vi "Main.vi"() -> ()   [LabVIEW 2020]
doc: "This template is for the Queued Message Handler design pattern.\n\nThe Event Handling Loop generates messages based on user interface actions.\n\nThe Message Handling Loop processes messages generated by the Event Handling Loop, or by other messages. The messages are string values, so new messages can be added easily to the Message Cases case structure in the Message Handling Loop. Each message cluster can also provide an optional value for Message Data, which is a variant that can be converted to whatever message-specific data is required."
uses:
  controls/WashIndicators.ctl
  controls/WashOptions.ctl
  controls/UI Data.ctl
  support/Message Queue/Message Queue.lvlib
  support/User Event - Stop/User Event - Stop.lvlib
panel:
  out "Wash Entry 2":bool
  in  "Wash Options":T1
  out "Car Wash Indicators 2":T2
  in  "Car Position Slider":u16(slide) scale=0.0..4.0
  out "Elapsed Time":dbl format="%<%H:%M:%S>t"
  in  "Start":bool
  in  "Stop":bool
  # "Pre-Soak\nH-P Wash\nL-P Wax\nSpot Free Rinse"
  # "Underbody Wash\nBug Remover"
  # "Tire Shine\nAir Dry"
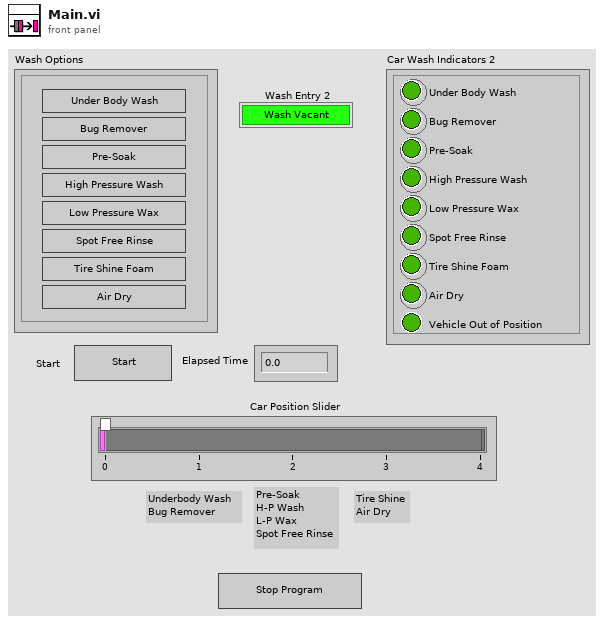
[diagram p1: front panel]
types:
  T1 = typedef "WashOptions.ctl" = cluster{"Bug Remover":bool, "Low Pressure Wax":bool, "High Pressure Wash":bool, "Pre-Soak":bool, "Spot Free Rinse":bool, "Air Dry":bool, "Under Body Wash":bool, "Tire Shine Foam":bool}
  T2 = typedef "WashIndicators.ctl" = cluster{"Bug Remover":bool, "Pre-Soak":bool, "High Pressure Wash":bool, "Spot Free Rinse":bool, "Tire Shine Foam":bool, "Low Pressure Wax":bool, "Vehicle Out of Position":bool, "Air Dry":bool, "Under Body Wash":bool}
  T3 = typedef "UI Data.ctl" = cluster{"Elapsed Time":refnum<vi>, "Car Position Slider":refnum<vi>, "Wash Options":refnum<vi>, "Car Wash Indicators 2":T2, "Wash Entry 2":bool}
  T4 = typedef "Message Queue.lvlib/All Message Queues.ctl" = cluster{"UI":refnum<queue>, "Status Loop":refnum<queue>}
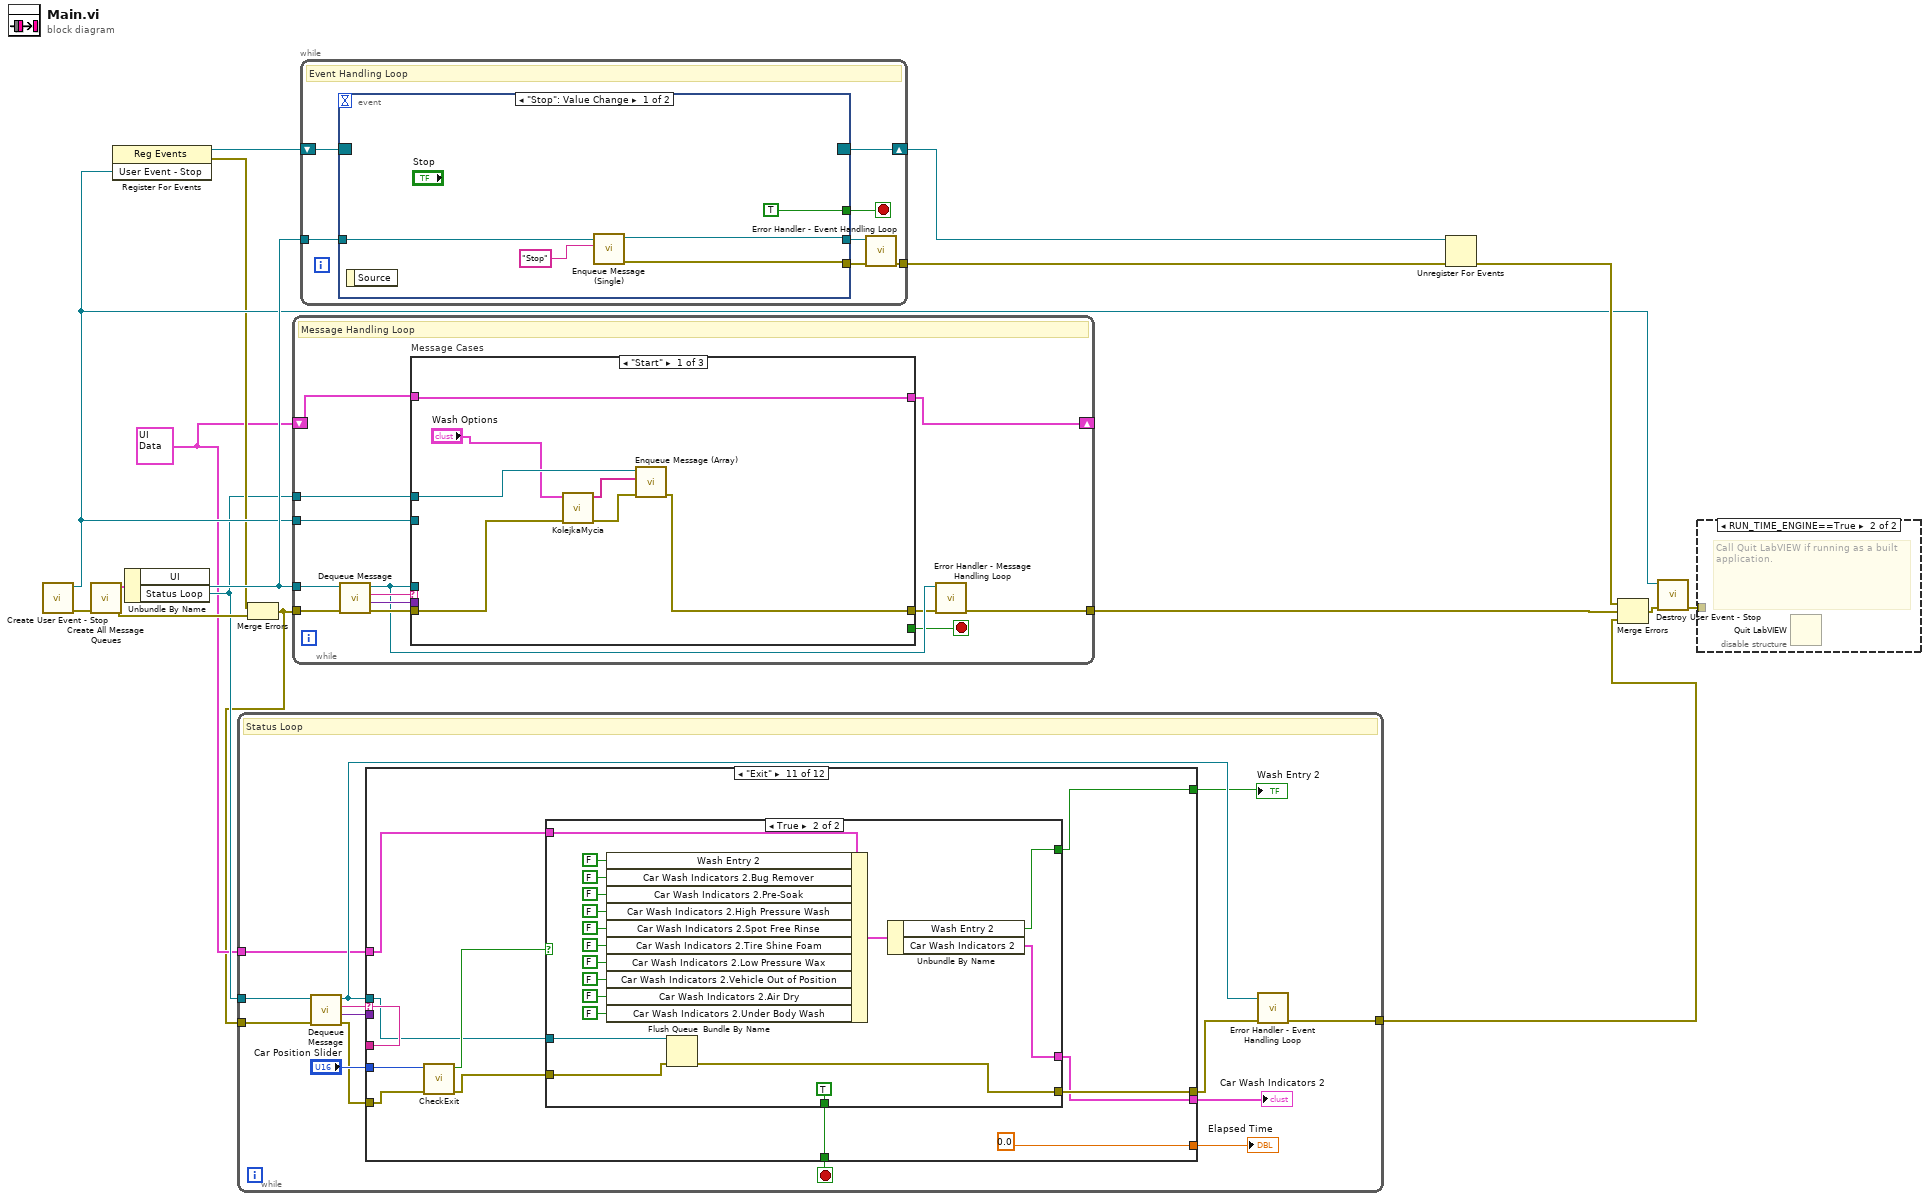
[diagram p0: block diagram]
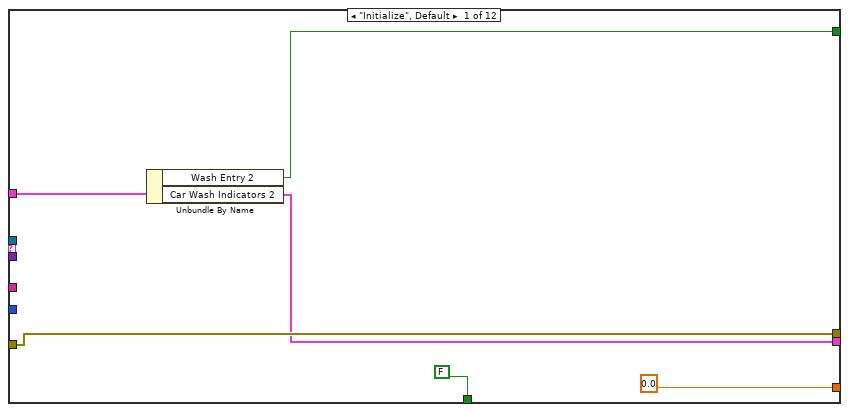
[diagram p2: hidden frame]
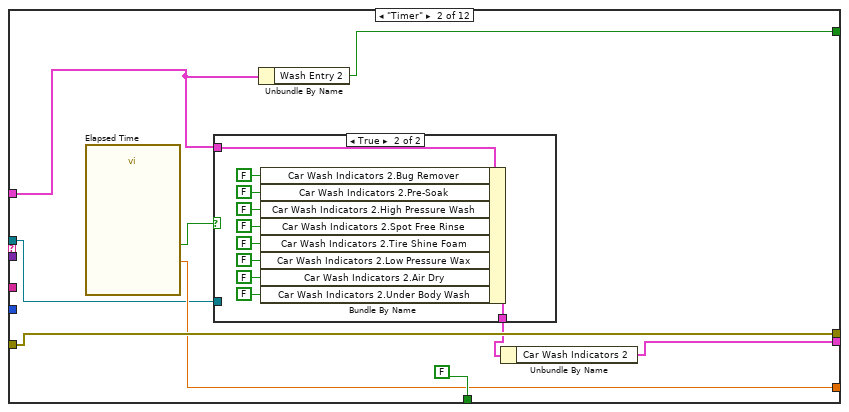
[diagram p3: hidden frame]
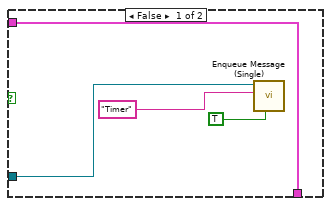
[diagram p4: hidden frame]
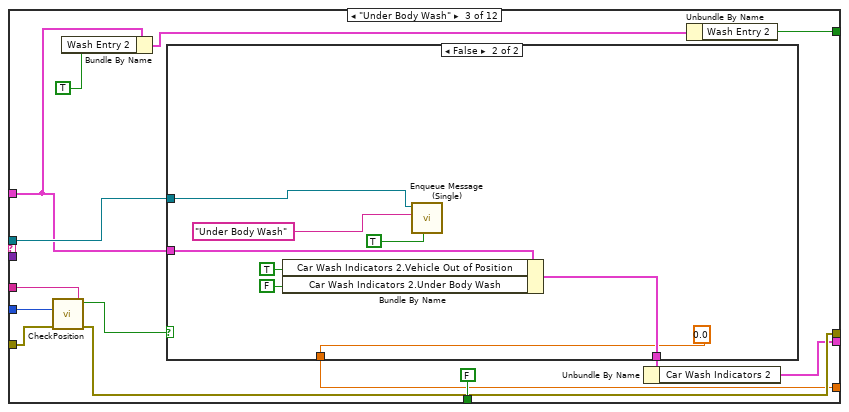
[diagram p5: hidden frame]
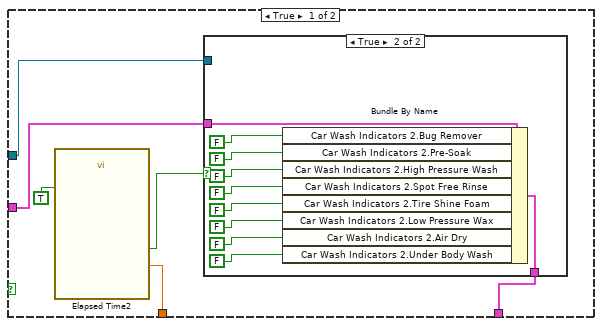
[diagram p6: hidden frame]
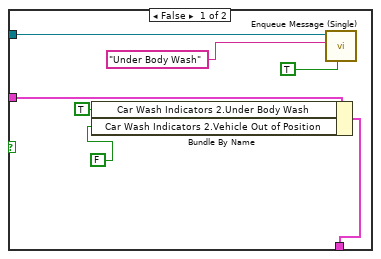
[diagram p7: hidden frame]
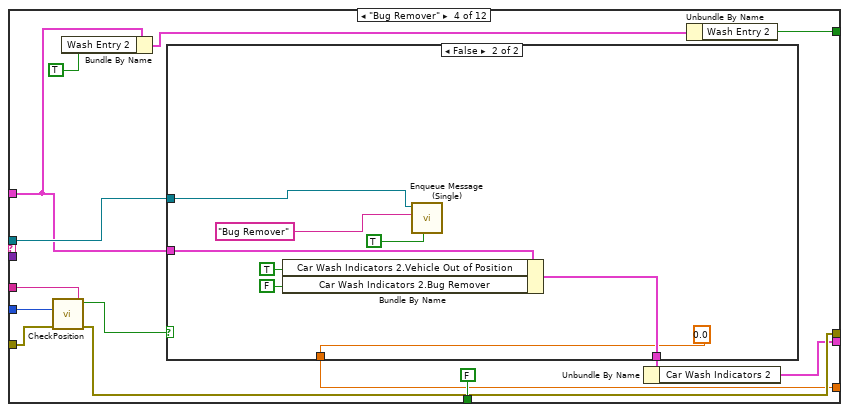
[diagram p8: hidden frame]
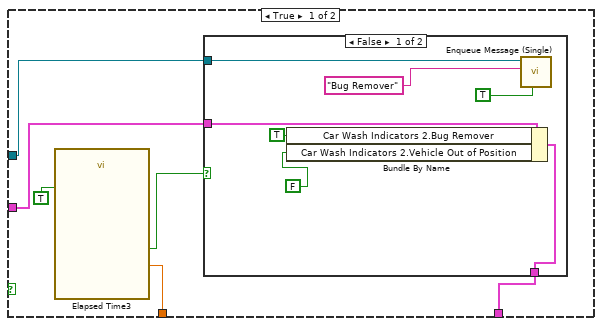
[diagram p9: hidden frame]
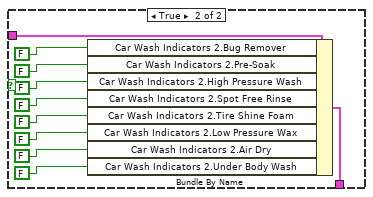
[diagram p10: hidden frame]
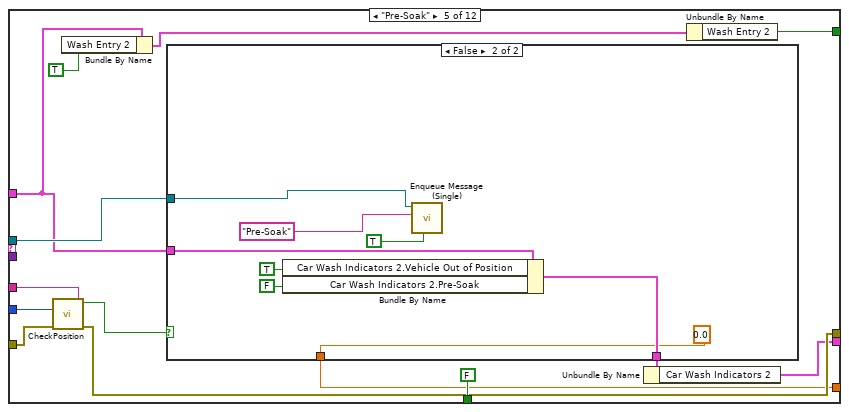
[diagram p11: hidden frame]
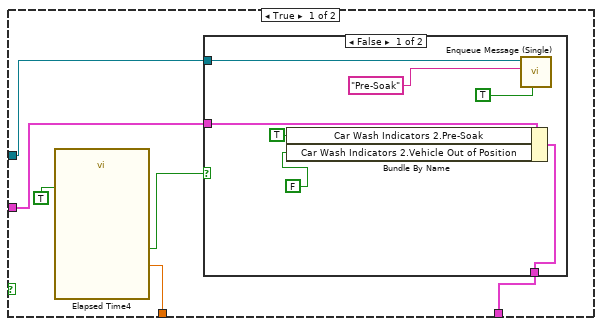
[diagram p12: hidden frame]
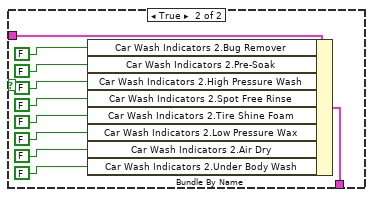
[diagram p13: hidden frame]
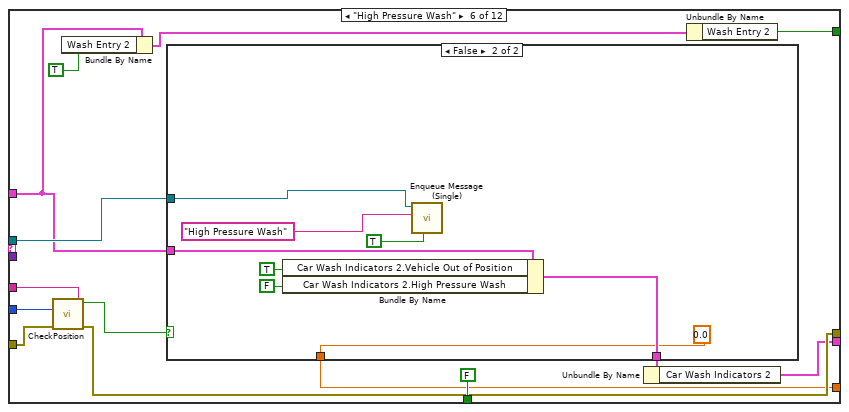
[diagram p14: hidden frame]
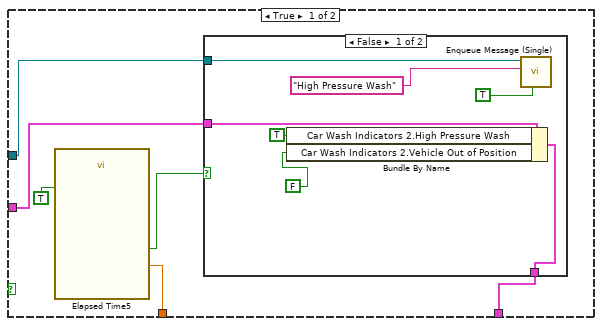
[diagram p15: hidden frame]
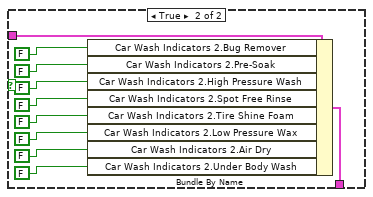
[diagram p16: hidden frame]
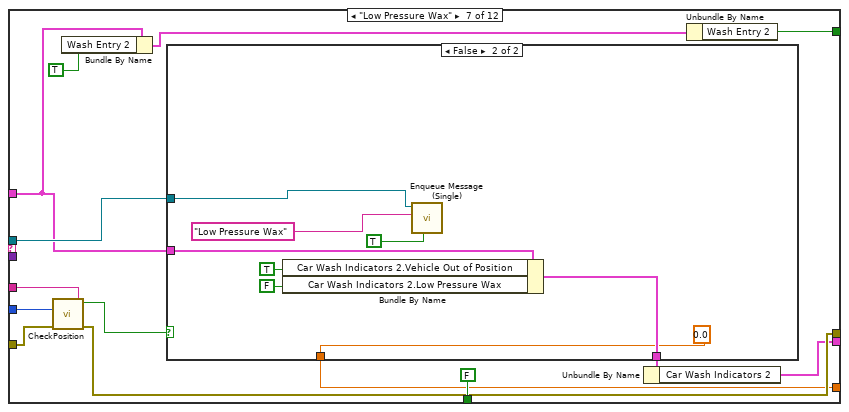
[diagram p17: hidden frame]
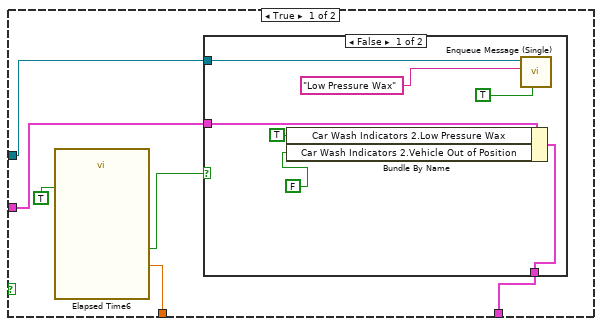
[diagram p18: hidden frame]
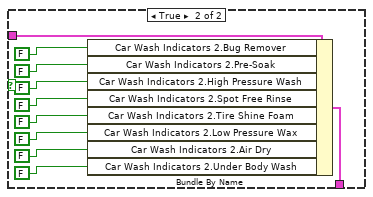
[diagram p19: hidden frame]
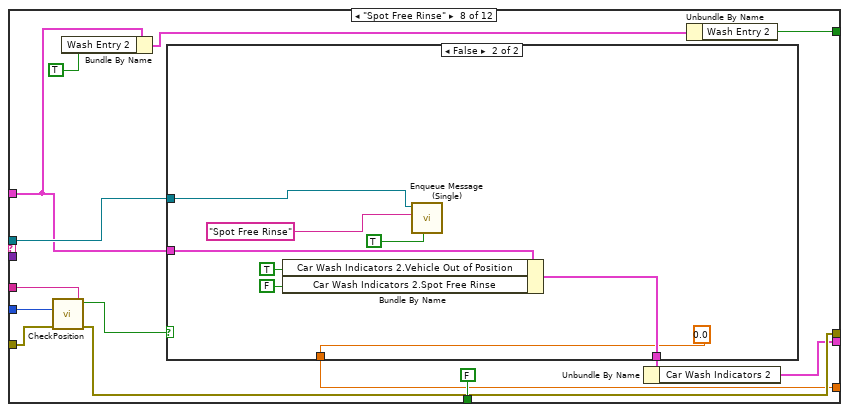
[diagram p20: hidden frame]
diagram:
  w2 = T3 {"Elapsed Time"=refnum, "Car Position Slider"=refnum, "Wash Options"=refnum, "Car Wash Indicators 2"={"Bug Remover"=FALSE, "Pre-Soak"=FALSE, "High Pressure Wash"=FALSE, "Spot Free Rinse"=FALSE, "Tire Shine Foam"=FALSE, "Low Pressure Wax"=FALSE, "Vehicle Out of Position"=FALSE, "Air Dry"=FALSE, "Under Body Wash"=FALSE}, "Wash Entry 2"=FALSE} ("Data Cluster")
  n1 = call "Create User Event - Stop.vi"() -> ("error out"=w13:errorcluster, "User Event - Stop"=w6:refnum<user-event>)  [unwired: 10 in]
  n2 = call "Create All Message Queues.vi"("error in (no error)"=w13) -> ("error out"=w17:errorcluster, "Message Queues out"=w16:T4)  [unwired: 9 in]
  n3 = register-events(w6) -> (reference out=w7:refnum<event-registration>, error out=w5:errorcluster)  [unwired: 2 in]
  n4 = Unbundle By Name(w16) -> ("UI"=w14:refnum<queue>, "Status Loop"=w3:refnum<queue>)
  n5 = Merge Errors(w5, w17) -> (w1:errorcluster)
  n6 = while {
    tunnel: w3 -> [w31]
    tunnel: w1 -> [w30]
    tunnel: [w27] -> w4
    tunnel: w2 -> [w25]
    stop <- w24 stop-if-true
    # "Status Loop"
    n7 = call "Dequeue Message.vi"("error in (no error)"=w30, "Message Queue"=w31) -> ("error out"=w21:errorcluster, "Message Data"=w29:variant, "Message"=w22:string, "dup Message Queue"=w26:refnum<queue>)  [unwired: 6 in]
    n8 = case shown="\"Exit\"" w22 {
      tunnel: w26 -> [_ w40 w69 w113 w158 w203 w248 w293 w338 w383 w425 w479]
      tunnel: w29 -> [_ _ _ _ _ _ _ _ _ _ _ _]
      tunnel: [w36 w45 w71 w115 w160 w205 w250 w295 w340 w385 w424 w482] -> w28
      tunnel: w25 -> [w35 w39 w65 w109 w154 w199 w244 w289 w334 w379 w423 w475]
      tunnel: [FALSE FALSE FALSE FALSE FALSE FALSE FALSE FALSE FALSE FALSE w426 TRUE] -> w24
      tunnel: "Car Position Slider" -> [_ _ w62 w117 w162 w207 w252 w297 w342 w387 w430 _]
      tunnel: w22 -> [_ _ w73 w118 w163 w208 w253 w298 w343 w388 _ _]
      tunnel: w21 -> [w36 w45 w72 w116 w161 w206 w251 w296 w341 w386 w429 w478]
      tunnel: [w34 w42 w67 w111 w156 w201 w246 w291 w336 w381 w421 w462] -> w20
      tunnel: [0.0 ("Elapsed Time (s)") w41 w66 w110 w155 w200 w245 w290 w335 w380 0.0 ("Elapsed Time (s)") 0.0 ("Elapsed Time (s)")] -> w19
      tunnel: [w32 w38 w63 w106 w151 w196 w241 w286 w331 w376 w422 w463] -> w18
      frame "Initialize", Default {
        n9 = Unbundle By Name(w35) -> ("Wash Entry 2"=w32:bool, "Car Wash Indicators 2"=w34:T2)
      }
      frame "Timer" {
        n10 = call "Elapsed Time"() -> ("Elapsed Time (s)"=w41:dbl, "Time has Elapsed"=w44:bool)  [unwired: 12 in, 6 out]
        n11 = case shown="True" w44 {
          tunnel: [w50 w52] -> w43
          tunnel: w39 -> [w50 w51]
          tunnel: w40 -> [w47 _]
          frame False {
            n12 = call "Enqueue Message (Single).vi"("Priority Message? (F)"=TRUE, "Message"="Timer", "Message Queue"=w47) -> ()  [unwired: 7 in, 2 out]
          }
          frame True {
            n13 = Bundle By Name(cluster=w51, "Car Wash Indicators 2.Bug Remover"=FALSE ("Bug Remover"), "Car Wash Indicators 2.Pre-Soak"=FALSE ("Pre-Soak"), "Car Wash Indicators 2.High Pressure Wash"=FALSE ("High Pressure Wash"), "Car Wash Indicators 2.Spot Free Rinse"=FALSE ("Spot Free Rinse"), "Car Wash Indicators 2.Tire Shine Foam"=FALSE ("Tire Shine Foam"), "Car Wash Indicators 2.Low Pressure Wax"=FALSE ("Low Pressure Wax"), "Car Wash Indicators 2.Air Dry"=FALSE ("Air Dry"), "Car Wash Indicators 2.Under Body Wash"=FALSE ("Under Body Wash")) -> (w52:T3)
          }
        }
        n14 = Unbundle By Name(w39) -> ("Wash Entry 2"=w38:bool)
        n15 = Unbundle By Name(w43) -> ("Car Wash Indicators 2"=w42:T2)
      }
      frame "Under Body Wash" {
        n16 = call "CheckPosition.vi"("error in"=w72, "Car Position"=w62, "State"=w73) -> ("error out"=w71:errorcluster, "Pozycja"=w70:bool)  [unwired: 7 in]
        n17 = Bundle By Name(cluster=w65, "Wash Entry 2"=TRUE) -> (w64:T3)
        n18 = case shown="False" w70 {
          tunnel: w65 -> [w76 w105]
          tunnel: w69 -> [w77 w102]
          tunnel: [w79 w99] -> w68
          tunnel: [w78 0.0 ("Elapsed Time (s)")] -> w66
          frame True {
            n19 = call "Elapsed Time2"("Auto Reset"=TRUE) -> ("Elapsed Time (s)"=w78:dbl, "Time has Elapsed"=w80:bool)  [unwired: 11 in, 6 out]
            n20 = case shown="True" w80 {
              tunnel: [w81 w89] -> w79
              tunnel: w77 -> [w85 _]
              tunnel: w76 -> [w84 w88]
              frame False {
                n21 = Bundle By Name(cluster=w84, "Car Wash Indicators 2.Under Body Wash"=TRUE, "Car Wash Indicators 2.Vehicle Out of Position"=FALSE) -> (w81:T3)
                n22 = call "Enqueue Message (Single).vi"("Priority Message? (F)"=TRUE, "Message"="Under Body Wash", "Message Queue"=w85) -> ()  [unwired: 7 in, 2 out]
              }
              frame True {
                n23 = Bundle By Name(cluster=w88, "Car Wash Indicators 2.Bug Remover"=FALSE ("Bug Remover"), "Car Wash Indicators 2.Pre-Soak"=FALSE ("Pre-Soak"), "Car Wash Indicators 2.High Pressure Wash"=FALSE ("High Pressure Wash"), "Car Wash Indicators 2.Spot Free Rinse"=FALSE ("Spot Free Rinse"), "Car Wash Indicators 2.Tire Shine Foam"=FALSE ("Tire Shine Foam"), "Car Wash Indicators 2.Low Pressure Wax"=FALSE ("Low Pressure Wax"), "Car Wash Indicators 2.Air Dry"=FALSE ("Air Dry"), "Car Wash Indicators 2.Under Body Wash"=FALSE ("Under Body Wash")) -> (w89:T3)
              }
            }
          }
          frame False {
            n24 = Bundle By Name(cluster=w105, "Car Wash Indicators 2.Vehicle Out of Position"=TRUE, "Car Wash Indicators 2.Under Body Wash"=FALSE) -> (w99:T3)
            n25 = call "Enqueue Message (Single).vi"("Priority Message? (F)"=TRUE, "Message"="Under Body Wash", "Message Queue"=w102) -> ()  [unwired: 7 in, 2 out]
          }
        }
        n26 = Unbundle By Name(w68) -> ("Car Wash Indicators 2"=w67:T2)
        n27 = Unbundle By Name(w64) -> ("Wash Entry 2"=w63:bool)
      }
      frame "Bug Remover" {
        n28 = call "CheckPosition.vi"("error in"=w116, "Car Position"=w117, "State"=w118) -> ("error out"=w115:errorcluster, "Pozycja"=w114:bool)  [unwired: 7 in]
        n29 = Bundle By Name(cluster=w109, "Wash Entry 2"=TRUE) -> (w107:T3)
        n30 = case shown="False" w114 {
          tunnel: w109 -> [w121 w150]
          tunnel: w113 -> [w122 w147]
          tunnel: [w124 w144] -> w112
          tunnel: [w123 0.0 ("Elapsed Time (s)")] -> w110
          frame True {
            n31 = call "Elapsed Time3"("Auto Reset"=TRUE) -> ("Elapsed Time (s)"=w123:dbl, "Time has Elapsed"=w125:bool)  [unwired: 11 in, 6 out]
            n32 = case shown="False" w125 {
              tunnel: [w126 w134] -> w124
              tunnel: w122 -> [w130 _]
              tunnel: w121 -> [w129 w133]
              frame False {
                n33 = Bundle By Name(cluster=w129, "Car Wash Indicators 2.Bug Remover"=TRUE ("Car Wash Indicators 2.Under Body Wash"), "Car Wash Indicators 2.Vehicle Out of Position"=FALSE) -> (w126:T3)
                n34 = call "Enqueue Message (Single).vi"("Priority Message? (F)"=TRUE, "Message"="Bug Remover", "Message Queue"=w130) -> ()  [unwired: 7 in, 2 out]
              }
              frame True {
                n35 = Bundle By Name(cluster=w133, "Car Wash Indicators 2.Bug Remover"=FALSE ("Bug Remover"), "Car Wash Indicators 2.Pre-Soak"=FALSE ("Pre-Soak"), "Car Wash Indicators 2.High Pressure Wash"=FALSE ("High Pressure Wash"), "Car Wash Indicators 2.Spot Free Rinse"=FALSE ("Spot Free Rinse"), "Car Wash Indicators 2.Tire Shine Foam"=FALSE ("Tire Shine Foam"), "Car Wash Indicators 2.Low Pressure Wax"=FALSE ("Low Pressure Wax"), "Car Wash Indicators 2.Air Dry"=FALSE ("Air Dry"), "Car Wash Indicators 2.Under Body Wash"=FALSE ("Under Body Wash")) -> (w134:T3)
              }
            }
          }
          frame False {
            n36 = Bundle By Name(cluster=w150, "Car Wash Indicators 2.Vehicle Out of Position"=TRUE, "Car Wash Indicators 2.Bug Remover"=FALSE ("Car Wash Indicators 2.Under Body Wash")) -> (w144:T3)
            n37 = call "Enqueue Message (Single).vi"("Priority Message? (F)"=TRUE, "Message"="Bug Remover", "Message Queue"=w147) -> ()  [unwired: 7 in, 2 out]
          }
        }
        n38 = Unbundle By Name(w112) -> ("Car Wash Indicators 2"=w111:T2)
        n39 = Unbundle By Name(w107) -> ("Wash Entry 2"=w106:bool)
      }
      frame "Pre-Soak" {
        n40 = call "CheckPosition.vi"("error in"=w161, "Car Position"=w162, "State"=w163) -> ("error out"=w160:errorcluster, "Pozycja"=w159:bool)  [unwired: 7 in]
        n41 = Bundle By Name(cluster=w154, "Wash Entry 2"=TRUE) -> (w152:T3)
        n42 = case shown="False" w159 {
          tunnel: w154 -> [w166 w195]
          tunnel: w158 -> [w167 w192]
          tunnel: [w169 w189] -> w157
          tunnel: [w168 0.0 ("Elapsed Time (s)")] -> w155
          frame True {
            n43 = call "Elapsed Time4"("Auto Reset"=TRUE) -> ("Elapsed Time (s)"=w168:dbl, "Time has Elapsed"=w170:bool)  [unwired: 11 in, 6 out]
            n44 = case shown="False" w170 {
              tunnel: [w171 w179] -> w169
              tunnel: w167 -> [w175 _]
              tunnel: w166 -> [w174 w178]
              frame False {
                n45 = Bundle By Name(cluster=w174, "Car Wash Indicators 2.Pre-Soak"=TRUE ("Car Wash Indicators 2.Under Body Wash"), "Car Wash Indicators 2.Vehicle Out of Position"=FALSE) -> (w171:T3)
                n46 = call "Enqueue Message (Single).vi"("Priority Message? (F)"=TRUE, "Message"="Pre-Soak", "Message Queue"=w175) -> ()  [unwired: 7 in, 2 out]
              }
              frame True {
                n47 = Bundle By Name(cluster=w178, "Car Wash Indicators 2.Bug Remover"=FALSE ("Bug Remover"), "Car Wash Indicators 2.Pre-Soak"=FALSE ("Pre-Soak"), "Car Wash Indicators 2.High Pressure Wash"=FALSE ("High Pressure Wash"), "Car Wash Indicators 2.Spot Free Rinse"=FALSE ("Spot Free Rinse"), "Car Wash Indicators 2.Tire Shine Foam"=FALSE ("Tire Shine Foam"), "Car Wash Indicators 2.Low Pressure Wax"=FALSE ("Low Pressure Wax"), "Car Wash Indicators 2.Air Dry"=FALSE ("Air Dry"), "Car Wash Indicators 2.Under Body Wash"=FALSE ("Under Body Wash")) -> (w179:T3)
              }
            }
          }
          frame False {
            n48 = Bundle By Name(cluster=w195, "Car Wash Indicators 2.Vehicle Out of Position"=TRUE, "Car Wash Indicators 2.Pre-Soak"=FALSE ("Car Wash Indicators 2.Under Body Wash")) -> (w189:T3)
            n49 = call "Enqueue Message (Single).vi"("Priority Message? (F)"=TRUE, "Message"="Pre-Soak", "Message Queue"=w192) -> ()  [unwired: 7 in, 2 out]
          }
        }
        n50 = Unbundle By Name(w157) -> ("Car Wash Indicators 2"=w156:T2)
        n51 = Unbundle By Name(w152) -> ("Wash Entry 2"=w151:bool)
      }
      frame "High Pressure Wash" {
        n52 = call "CheckPosition.vi"("error in"=w206, "Car Position"=w207, "State"=w208) -> ("error out"=w205:errorcluster, "Pozycja"=w204:bool)  [unwired: 7 in]
        n53 = Bundle By Name(cluster=w199, "Wash Entry 2"=TRUE) -> (w197:T3)
        n54 = case shown="False" w204 {
          tunnel: w199 -> [w211 w240]
          tunnel: w203 -> [w212 w237]
          tunnel: [w214 w234] -> w202
          tunnel: [w213 0.0 ("Elapsed Time (s)")] -> w200
          frame True {
            n55 = call "Elapsed Time5"("Auto Reset"=TRUE) -> ("Elapsed Time (s)"=w213:dbl, "Time has Elapsed"=w215:bool)  [unwired: 11 in, 6 out]
            n56 = case shown="False" w215 {
              tunnel: [w216 w224] -> w214
              tunnel: w212 -> [w220 _]
              tunnel: w211 -> [w219 w223]
              frame False {
                n57 = Bundle By Name(cluster=w219, "Car Wash Indicators 2.High Pressure Wash"=TRUE ("Car Wash Indicators 2.Under Body Wash"), "Car Wash Indicators 2.Vehicle Out of Position"=FALSE) -> (w216:T3)
                n58 = call "Enqueue Message (Single).vi"("Priority Message? (F)"=TRUE, "Message"="High Pressure Wash", "Message Queue"=w220) -> ()  [unwired: 7 in, 2 out]
              }
              frame True {
                n59 = Bundle By Name(cluster=w223, "Car Wash Indicators 2.Bug Remover"=FALSE ("Bug Remover"), "Car Wash Indicators 2.Pre-Soak"=FALSE ("Pre-Soak"), "Car Wash Indicators 2.High Pressure Wash"=FALSE ("High Pressure Wash"), "Car Wash Indicators 2.Spot Free Rinse"=FALSE ("Spot Free Rinse"), "Car Wash Indicators 2.Tire Shine Foam"=FALSE ("Tire Shine Foam"), "Car Wash Indicators 2.Low Pressure Wax"=FALSE ("Low Pressure Wax"), "Car Wash Indicators 2.Air Dry"=FALSE ("Air Dry"), "Car Wash Indicators 2.Under Body Wash"=FALSE ("Under Body Wash")) -> (w224:T3)
              }
            }
          }
          frame False {
            n60 = Bundle By Name(cluster=w240, "Car Wash Indicators 2.Vehicle Out of Position"=TRUE, "Car Wash Indicators 2.High Pressure Wash"=FALSE ("Car Wash Indicators 2.Under Body Wash")) -> (w234:T3)
            n61 = call "Enqueue Message (Single).vi"("Priority Message? (F)"=TRUE, "Message"="High Pressure Wash", "Message Queue"=w237) -> ()  [unwired: 7 in, 2 out]
          }
        }
        n62 = Unbundle By Name(w202) -> ("Car Wash Indicators 2"=w201:T2)
        n63 = Unbundle By Name(w197) -> ("Wash Entry 2"=w196:bool)
      }
      frame "Low Pressure Wax" {
        n64 = call "CheckPosition.vi"("error in"=w251, "Car Position"=w252, "State"=w253) -> ("error out"=w250:errorcluster, "Pozycja"=w249:bool)  [unwired: 7 in]
        n65 = Bundle By Name(cluster=w244, "Wash Entry 2"=TRUE) -> (w242:T3)
        n66 = case shown="False" w249 {
          tunnel: w244 -> [w256 w285]
          tunnel: w248 -> [w257 w282]
          tunnel: [w259 w279] -> w247
          tunnel: [w258 0.0 ("Elapsed Time (s)")] -> w245
          frame True {
            n67 = call "Elapsed Time6"("Auto Reset"=TRUE) -> ("Elapsed Time (s)"=w258:dbl, "Time has Elapsed"=w260:bool)  [unwired: 11 in, 6 out]
            n68 = case shown="False" w260 {
              tunnel: [w261 w269] -> w259
              tunnel: w257 -> [w265 _]
              tunnel: w256 -> [w264 w268]
              frame False {
                n69 = Bundle By Name(cluster=w264, "Car Wash Indicators 2.Low Pressure Wax"=TRUE ("Car Wash Indicators 2.Under Body Wash"), "Car Wash Indicators 2.Vehicle Out of Position"=FALSE) -> (w261:T3)
                n70 = call "Enqueue Message (Single).vi"("Priority Message? (F)"=TRUE, "Message"="Low Pressure Wax", "Message Queue"=w265) -> ()  [unwired: 7 in, 2 out]
              }
              frame True {
                n71 = Bundle By Name(cluster=w268, "Car Wash Indicators 2.Bug Remover"=FALSE ("Bug Remover"), "Car Wash Indicators 2.Pre-Soak"=FALSE ("Pre-Soak"), "Car Wash Indicators 2.High Pressure Wash"=FALSE ("High Pressure Wash"), "Car Wash Indicators 2.Spot Free Rinse"=FALSE ("Spot Free Rinse"), "Car Wash Indicators 2.Tire Shine Foam"=FALSE ("Tire Shine Foam"), "Car Wash Indicators 2.Low Pressure Wax"=FALSE ("Low Pressure Wax"), "Car Wash Indicators 2.Air Dry"=FALSE ("Air Dry"), "Car Wash Indicators 2.Under Body Wash"=FALSE ("Under Body Wash")) -> (w269:T3)
              }
            }
          }
          frame False {
            n72 = Bundle By Name(cluster=w285, "Car Wash Indicators 2.Vehicle Out of Position"=TRUE, "Car Wash Indicators 2.Low Pressure Wax"=FALSE ("Car Wash Indicators 2.Under Body Wash")) -> (w279:T3)
            n73 = call "Enqueue Message (Single).vi"("Priority Message? (F)"=TRUE, "Message"="Low Pressure Wax", "Message Queue"=w282) -> ()  [unwired: 7 in, 2 out]
          }
        }
        n74 = Unbundle By Name(w247) -> ("Car Wash Indicators 2"=w246:T2)
        n75 = Unbundle By Name(w242) -> ("Wash Entry 2"=w241:bool)
      }
      frame "Spot Free Rinse" {
        n76 = call "CheckPosition.vi"("error in"=w296, "Car Position"=w297, "State"=w298) -> ("error out"=w295:errorcluster, "Pozycja"=w294:bool)  [unwired: 7 in]
        n77 = Bundle By Name(cluster=w289, "Wash Entry 2"=TRUE) -> (w287:T3)
        n78 = case shown="False" w294 {
          tunnel: w289 -> [w301 w330]
          tunnel: w293 -> [w302 w327]
          tunnel: [w304 w324] -> w292
          tunnel: [w303 0.0 ("Elapsed Time (s)")] -> w290
          frame True {
            n79 = call "Elapsed Time7"("Auto Reset"=TRUE) -> ("Elapsed Time (s)"=w303:dbl, "Time has Elapsed"=w305:bool)  [unwired: 11 in, 6 out]
            n80 = case shown="False" w305 {
              tunnel: [w306 w314] -> w304
              tunnel: w302 -> [w310 _]
              tunnel: w301 -> [w309 w313]
              frame False {
                n81 = Bundle By Name(cluster=w309, "Car Wash Indicators 2.Spot Free Rinse"=TRUE ("Car Wash Indicators 2.Under Body Wash"), "Car Wash Indicators 2.Vehicle Out of Position"=FALSE) -> (w306:T3)
                n82 = call "Enqueue Message (Single).vi"("Priority Message? (F)"=TRUE, "Message"="Spot Free Rinse", "Message Queue"=w310) -> ()  [unwired: 7 in, 2 out]
              }
              frame True {
                n83 = Bundle By Name(cluster=w313, "Car Wash Indicators 2.Bug Remover"=FALSE ("Bug Remover"), "Car Wash Indicators 2.Pre-Soak"=FALSE ("Pre-Soak"), "Car Wash Indicators 2.High Pressure Wash"=FALSE ("High Pressure Wash"), "Car Wash Indicators 2.Spot Free Rinse"=FALSE ("Spot Free Rinse"), "Car Wash Indicators 2.Tire Shine Foam"=FALSE ("Tire Shine Foam"), "Car Wash Indicators 2.Low Pressure Wax"=FALSE ("Low Pressure Wax"), "Car Wash Indicators 2.Air Dry"=FALSE ("Air Dry"), "Car Wash Indicators 2.Under Body Wash"=FALSE ("Under Body Wash")) -> (w314:T3)
              }
            }
          }
          frame False {
            n84 = Bundle By Name(cluster=w330, "Car Wash Indicators 2.Vehicle Out of Position"=TRUE, "Car Wash Indicators 2.Spot Free Rinse"=FALSE ("Car Wash Indicators 2.Under Body Wash")) -> (w324:T3)
            n85 = call "Enqueue Message (Single).vi"("Priority Message? (F)"=TRUE, "Message"="Spot Free Rinse", "Message Queue"=w327) -> ()  [unwired: 7 in, 2 out]
          }
        }
        n86 = Unbundle By Name(w292) -> ("Car Wash Indicators 2"=w291:T2)
        n87 = Unbundle By Name(w287) -> ("Wash Entry 2"=w286:bool)
      }
      frame "Tire Shine Foam" {
        n88 = call "CheckPosition.vi"("error in"=w341, "Car Position"=w342, "State"=w343) -> ("error out"=w340:errorcluster, "Pozycja"=w339:bool)  [unwired: 7 in]
        n89 = Bundle By Name(cluster=w334, "Wash Entry 2"=TRUE) -> (w332:T3)
        n90 = case shown="False" w339 {
          tunnel: w334 -> [w346 w375]
          tunnel: w338 -> [w347 w372]
          tunnel: [w349 w369] -> w337
          tunnel: [w348 0.0 ("Elapsed Time (s)")] -> w335
          frame True {
            n91 = call "Elapsed Time8"("Auto Reset"=TRUE) -> ("Elapsed Time (s)"=w348:dbl, "Time has Elapsed"=w350:bool)  [unwired: 11 in, 6 out]
            n92 = case shown="False" w350 {
              tunnel: [w351 w359] -> w349
              tunnel: w347 -> [w355 _]
              tunnel: w346 -> [w354 w358]
              frame False {
                n93 = Bundle By Name(cluster=w354, "Car Wash Indicators 2.Tire Shine Foam"=TRUE ("Car Wash Indicators 2.Under Body Wash"), "Car Wash Indicators 2.Vehicle Out of Position"=FALSE) -> (w351:T3)
                n94 = call "Enqueue Message (Single).vi"("Priority Message? (F)"=TRUE, "Message"="Tire Shine Foam", "Message Queue"=w355) -> ()  [unwired: 7 in, 2 out]
              }
              frame True {
                n95 = Bundle By Name(cluster=w358, "Car Wash Indicators 2.Bug Remover"=FALSE ("Bug Remover"), "Car Wash Indicators 2.Pre-Soak"=FALSE ("Pre-Soak"), "Car Wash Indicators 2.High Pressure Wash"=FALSE ("High Pressure Wash"), "Car Wash Indicators 2.Spot Free Rinse"=FALSE ("Spot Free Rinse"), "Car Wash Indicators 2.Tire Shine Foam"=FALSE ("Tire Shine Foam"), "Car Wash Indicators 2.Low Pressure Wax"=FALSE ("Low Pressure Wax"), "Car Wash Indicators 2.Air Dry"=FALSE ("Air Dry"), "Car Wash Indicators 2.Under Body Wash"=FALSE ("Under Body Wash")) -> (w359:T3)
              }
            }
          }
          frame False {
            n96 = Bundle By Name(cluster=w375, "Car Wash Indicators 2.Vehicle Out of Position"=TRUE, "Car Wash Indicators 2.Tire Shine Foam"=FALSE ("Car Wash Indicators 2.Under Body Wash")) -> (w369:T3)
            n97 = call "Enqueue Message (Single).vi"("Priority Message? (F)"=TRUE, "Message"="Tire Shine Foam", "Message Queue"=w372) -> ()  [unwired: 7 in, 2 out]
          }
        }
        n98 = Unbundle By Name(w337) -> ("Car Wash Indicators 2"=w336:T2)
        n99 = Unbundle By Name(w332) -> ("Wash Entry 2"=w331:bool)
      }
      frame "Air Dry" {
        n100 = call "CheckPosition.vi"("error in"=w386, "Car Position"=w387, "State"=w388) -> ("error out"=w385:errorcluster, "Pozycja"=w384:bool)  [unwired: 7 in]
        n101 = Bundle By Name(cluster=w379, "Wash Entry 2"=TRUE) -> (w377:T3)
        n102 = case shown="False" w384 {
          tunnel: w379 -> [w391 w420]
          tunnel: w383 -> [w392 w417]
          tunnel: [w394 w414] -> w382
          tunnel: [w393 0.0 ("Elapsed Time (s)")] -> w380
          frame True {
            n103 = call "Elapsed Time9"("Auto Reset"=TRUE) -> ("Elapsed Time (s)"=w393:dbl, "Time has Elapsed"=w395:bool)  [unwired: 11 in, 6 out]
            n104 = case shown="True" w395 {
              tunnel: [w396 w404] -> w394
              tunnel: w392 -> [w400 _]
              tunnel: w391 -> [w399 w403]
              frame False {
                n105 = Bundle By Name(cluster=w399, "Car Wash Indicators 2.Air Dry"=TRUE ("Car Wash Indicators 2.Under Body Wash"), "Car Wash Indicators 2.Vehicle Out of Position"=FALSE) -> (w396:T3)
                n106 = call "Enqueue Message (Single).vi"("Priority Message? (F)"=TRUE, "Message"="Air Dry", "Message Queue"=w400) -> ()  [unwired: 7 in, 2 out]
              }
              frame True {
                n107 = Bundle By Name(cluster=w403, "Car Wash Indicators 2.Bug Remover"=FALSE ("Bug Remover"), "Car Wash Indicators 2.Pre-Soak"=FALSE ("Pre-Soak"), "Car Wash Indicators 2.High Pressure Wash"=FALSE ("High Pressure Wash"), "Car Wash Indicators 2.Spot Free Rinse"=FALSE ("Spot Free Rinse"), "Car Wash Indicators 2.Tire Shine Foam"=FALSE ("Tire Shine Foam"), "Car Wash Indicators 2.Low Pressure Wax"=FALSE ("Low Pressure Wax"), "Car Wash Indicators 2.Air Dry"=FALSE ("Air Dry"), "Car Wash Indicators 2.Under Body Wash"=FALSE ("Under Body Wash")) -> (w404:T3)
              }
            }
          }
          frame False {
            n108 = Bundle By Name(cluster=w420, "Car Wash Indicators 2.Vehicle Out of Position"=TRUE, "Car Wash Indicators 2.Air Dry"=FALSE ("Car Wash Indicators 2.Under Body Wash")) -> (w414:T3)
            n109 = call "Enqueue Message (Single).vi"("Priority Message? (F)"=TRUE, "Message"="Air Dry", "Message Queue"=w417) -> ()  [unwired: 7 in, 2 out]
          }
        }
        n110 = Unbundle By Name(w382) -> ("Car Wash Indicators 2"=w381:T2)
        n111 = Unbundle By Name(w377) -> ("Wash Entry 2"=w376:bool)
      }
      frame "Exit" {
        n112 = call "CheckExit.vi"("error in"=w429, "Car Position Slider"=w430) -> ("error out"=w427:errorcluster, "check"=w428:bool)  [unwired: 8 in]
        n113 = case shown="True" w428 {
          tunnel: w427 -> [w435 w448]
          tunnel: [FALSE TRUE] -> w426
          tunnel: w425 -> [w436 w449]
          tunnel: [w434 w444] -> w424
          tunnel: w423 -> [w443 w447]
          tunnel: [w440 w446] -> w422
          tunnel: [w439 w445] -> w421
          frame False {
            n114 = Bundle By Name(cluster=w443, "Car Wash Indicators 2.Vehicle Out of Position"=TRUE, "Wash Entry 2"=TRUE) -> (w441:T3)
            n115 = call "Enqueue Message (Single).vi"("Priority Message? (F)"=TRUE, "error in (no error)"=w435, "Message"="Exit", "Message Queue"=w436) -> ("error out"=w434:errorcluster)  [unwired: 6 in, 1 out]
            n116 = Unbundle By Name(w441) -> ("Wash Entry 2"=w440:bool, "Car Wash Indicators 2"=w439:T2)
          }
          frame True {
            n117 = Bundle By Name(cluster=w447, "Wash Entry 2"=FALSE, "Car Wash Indicators 2.Bug Remover"=FALSE, "Car Wash Indicators 2.Pre-Soak"=FALSE, "Car Wash Indicators 2.High Pressure Wash"=FALSE, "Car Wash Indicators 2.Spot Free Rinse"=FALSE, "Car Wash Indicators 2.Tire Shine Foam"=FALSE, "Car Wash Indicators 2.Low Pressure Wax"=FALSE, "Car Wash Indicators 2.Vehicle Out of Position"=FALSE, "Car Wash Indicators 2.Air Dry"=FALSE, "Car Wash Indicators 2.Under Body Wash"=FALSE) -> (w460:T3)
            n118 = Flush Queue(queue=w449, error in (no error)=w448) -> (error out=w444:errorcluster)  [unwired: 2 out]
            n119 = Unbundle By Name(w460) -> ("Wash Entry 2"=w446:bool, "Car Wash Indicators 2"=w445:T2)
          }
        }
      }
      frame "Stop" {
        n120 = Flush Queue(queue=w479, error in (no error)=w478) -> (queue out=w476:refnum<queue>, error out=w477:errorcluster)  [unwired: 1 out]
        n121 = Release Queue(queue=w476, error in (no error)=w477) -> (error out=w482:errorcluster)  [unwired: 1 in, 2 out]
        n122 = Bundle By Name(cluster=w475, "Wash Entry 2"=FALSE, "Car Wash Indicators 2.Bug Remover"=FALSE, "Car Wash Indicators 2.Pre-Soak"=FALSE, "Car Wash Indicators 2.High Pressure Wash"=FALSE, "Car Wash Indicators 2.Spot Free Rinse"=FALSE, "Car Wash Indicators 2.Tire Shine Foam"=FALSE, "Car Wash Indicators 2.Low Pressure Wax"=FALSE, "Car Wash Indicators 2.Vehicle Out of Position"=FALSE, "Car Wash Indicators 2.Air Dry"=FALSE, "Car Wash Indicators 2.Under Body Wash"=FALSE) -> (w464:T3)
        n123 = Unbundle By Name(w464) -> ("Wash Entry 2"=w463:bool, "Car Wash Indicators 2"=w462:T2)
      }
    }
    "Car Wash Indicators 2" <- w20
    "Elapsed Time" <- w19
    "Wash Entry 2" <- w18
    n124 = call "Error Handler - Event Handling Loop.vi"("error in (no error)"=w28, "Message Queue"=w26) -> ("dup error in"=w27:errorcluster)  [unwired: 8 in, 1 out]
  }
  n125 = while {
    tunnel: w14 -> [w489]
    shift-right: [w483] -> _
    shift-left: w2 -> [w495]
    tunnel: w6 -> [w494]
    tunnel: w1 -> [w493]
    tunnel: [w487] -> w15
    tunnel: w3 -> [w484]
    stop <- w485 stop-if-true
    # "Message Handling Loop"
    n126 = call "Dequeue Message.vi"("error in (no error)"=w493, "Message Queue"=w489) -> ("error out"=w492:errorcluster, "Message Data"=w490:variant, "Message"=w491:string, "dup Message Queue"=w488:refnum<queue>)  [unwired: 6 in]
    n127 = case "Message Cases" shown="\"Start\"" w491 {
      tunnel: w488 -> [_ _ w519]
      tunnel: w492 -> [w502 w506 w521]
      tunnel: [w497 w506 w522] -> w486
      tunnel: w495 -> [w498 w508 w509]
      tunnel: [w498 w507 w509] -> w483
      tunnel: [_ _ TRUE] -> w485
      tunnel: w490 -> [_ _ w513]
      tunnel: w494 -> [_ _ w514]
      tunnel: w484 -> [w501 _ w518]
      frame "Start" {
        # "Initialize - All initialization work should take place in this message, since other loops can potentially enqueue messages that execute immediately after this one."
        n128 = call "KolejkaMycia.vi"("error in (no error)"=w502, "Wash Options"="Wash Options") -> ("error out"=w499:errorcluster, "Option Array"=w500:string[])  [unwired: 8 in]
        n129 = call "Enqueue Message (Array).vi"("error in (no error)"=w499, "Message Array"=w500, "Message Queue"=w501) -> ("error out"=w497:errorcluster)  [unwired: 7 in, 1 out]
      }
      frame "Initialize", Default {
        # "Initialize - All initialization work should take place in this message, since other loops can potentially enqueue messages that execute immediately after this one."
        n130 = control-ref of="Wash Options"() -> (w503:refnum<vi>)
        n131 = control-ref of="Elapsed Time"() -> (w505:refnum<vi>)
        n132 = control-ref of="Car Position Slider"() -> (w504:refnum<vi>)
        n133 = Bundle By Name(cluster=w508, "Wash Options"=w503, "Elapsed Time"=w505, "Car Position Slider"=w504) -> (w507:T3)
      }
      frame "Stop" {
        # "Something - Replace this message with functionality for your own application."
        n134 = call-poly "Enqueue Message.vi"("Priority Message? (F)"=TRUE, "error in (no error)"=w521, "Message"="Stop", "Message Queue"=w518) -> ("error out"=w520:errorcluster)  [unwired: 6 in, 1 out]
        n135 = Release Queue(queue=w519, error in (no error)=w520) -> (error out=w516:errorcluster)  [unwired: 1 in, 2 out]
        n136 = Variant To Data(Variant=w513) -> (data=w512:errorcluster)  [unwired: 2 in, 1 out]
        n137 = call <vilib>:"Simple Error Handler.vi"("error in (no error)"=w512) -> ()  [unwired: 4 in, 5 out]
        n138 = call "Fire User Event - Stop.vi"("User Event - Stop"=w514) -> ("error out"=w515:errorcluster)  [unwired: 10 in]
        n139 = Merge Errors(w515, w516) -> (w522:errorcluster)
      }
    }
    n140 = call "Error Handler - Message Handling Loop.vi"("error in (no error)"=w486, "Message Queue"=w488) -> ("dup error in"=w487:errorcluster)  [unwired: 8 in, 1 out]
  }
  n141 = while {
    tunnel: w14 -> [w529]
    shift-right: [w527] -> w10
    shift-left: w7 -> [w528]
    tunnel: [w525] -> w8
    stop <- w523 stop-if-true
    # "Event Handling Loop"
    n142 = event shown="[0] \"Stop\": Value Change" {
      selector: w528 -> [_ _]
      dyn-events: [_ _] -> w527
      timeout: _ -> [_ _]
      tunnel: w529 -> [w534 w537]
      tunnel: [w533 w535] -> w526
      tunnel: [w531 w536] -> w524
      tunnel: [TRUE _] -> w523
      event "Stop": Value Change {
        n143 = event-data() -> ()  [unwired: 1 in, 1 out]
        n144 = call "Enqueue Message (Single).vi"("Message"="Stop", "Message Queue"=w534) -> ("error out"=w531:errorcluster, "dup Message Queue"=w533:refnum<queue>)  [unwired: 8 in]
      }
      event "Start": Value Change {
        n145 = event-data() -> ()  [unwired: 1 in, 1 out]
        n146 = call-poly "Enqueue Message.vi"("Message"="Start", "Message Queue"=w537) -> ("error out"=w536:errorcluster, "dup Message Queue"=w535:refnum<queue>)  [unwired: 8 in]
      }
    }
    n147 = call "Error Handler - Event Handling Loop.vi"("error in (no error)"=w524, "Message Queue"=w526) -> ("dup error in"=w525:errorcluster)  [unwired: 8 in, 1 out]
  }
  n148 = Unregister For Events(event registration refnum=w10, error in=w8) -> (error out=w11:errorcluster)
  n149 = Merge Errors(w11, w15, w4) -> (w12:errorcluster)
  n150 = call "Destroy User Event - Stop.vi"("error in (no error)"=w12, "User Event - Stop"=w6) -> ("error out"=w9:errorcluster)  [unwired: 9 in]
  n151 = disable-structure shown="RUN_TIME_ENGINE==True" {
    disable-tunnel: w9 -> [_ _]
    frame condition #0 (active) {
    }
    frame condition #1 {
      # "Call Quit LabVIEW if running as a built application."
      n152 = Quit LabVIEW() -> ()  [unwired: 1 in]
    }
  }
